vi "Create Parent Folder.vi"(10 "Accessor Options":T1, 11 "LVClassLibrary":refnum<vi>) -> (2 "Item Name":string, 3 "Parent":refnum<vi>)   [LabVIEW 2018, in "LVClassByRef.lvlib"]
uses:
  <resource>/Framework/Providers/LVClassByRef/LVClassByRef.lvlib
  <resource>/Framework/Providers/LVClassByRef/Accessor Options.ctl
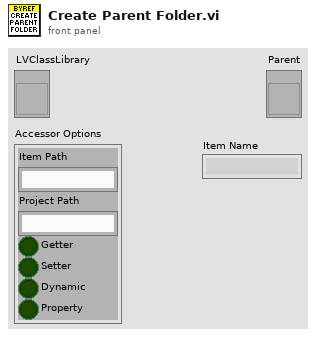
[diagram p1: front panel]
types:
  T1 = typedef "LVClassByRef.lvlib/Accessor Options.ctl" = cluster{"Item Path":string, "Project Path":string, "Getter":bool, "Setter":bool, "Dynamic":bool, "Property":bool}
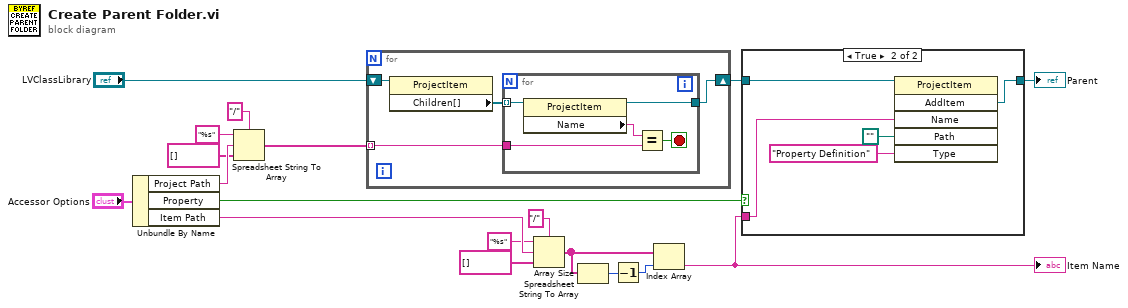
[diagram p0: block diagram]
diagram:
  n1 = Unbundle By Name("Accessor Options") -> ("Project Path"=w17:string, "Property"=w11:bool, "Item Path"=w9:string)
  n2 = Spreadsheet String To Array(delimiter (Tab)="/", format string="%s", spreadsheet string=w17, array type (2D Dbl)=string[] []) -> (array=w13:string[])
  n3 = for {
    tunnel: w13 -> [w21] mode=indexing
    shift-right: [w19] -> w10
    shift-left: "LVClassLibrary" -> [w22]
    n4 = property class="ProjectItem"(reference=w22) -> ("Children[]"=w20:refnum<vi>[])  [unwired: 1 in, 2 out]
    n5 = for {
      tunnel: w21 -> [w25]
      tunnel: w20 -> [w27] mode=indexing
      tunnel: [w23] -> w19
      stop <- w24 stop-if-true
      n6 = property class="ProjectItem"(reference=w27) -> (reference out=w23:refnum<vi>, "Name"=w26:string)  [unwired: 1 in, 1 out]
      n7 = Equal?(x=w26, y=w25) -> (x = y?=w24:bool)
    }
  }
  n8 = Spreadsheet String To Array(delimiter (Tab)="/", format string="%s", spreadsheet string=w9, array type (2D Dbl)=string[] []) -> (array=w6:string[])
  n9 = Array Size(array=w6) -> (size(s)=w5:i32)
  n10 = Decrement(x=w5) -> (x-1=w7:i32)
  n11 = Index Array(array=w6, index=w7) -> (element=w1:string)
  "Item Name" <- w1
  n12 = case shown="True" w11 {
    tunnel: w10 -> [w28 w33]
    tunnel: [w28 w31] -> w8
    tunnel: w1 -> [_ w29]
    frame False {
    }
    frame True {
      n13 = invoke class="ProjectItem" method="AddItem"(reference=w33, "Name"=w29, "Path"=path "", "Type"="Property Definition") -> ("AddItem"=w31:refnum<vi>)  [unwired: 2 in, 5 out]
    }
  }
  "Parent" <- w8
